vi "Test Configure device.vi"   [LabVIEW 2020]
uses:
  WS1051 1.1/WS1051 1.1.lvclass
  C:/Sandbox/RF Bench/Source Code/WiSpry Test Framework/Devices/Toggle 7/Toggle 7.1.lvclass
  WS1050 1.1/WS1050 1.1.lvclass
  Controls/Change setting mode enum.ctl
  Toggle 7.1.lvclass
  PIC-device/PIC-Device.lvclass
types:
  T1 = typedef "PIC-Device.lvclass/Change setting mode enum.ctl" = enum16{"Init", "Next", "Reset"}
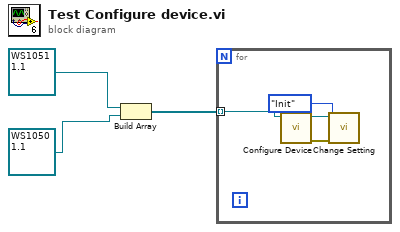
[diagram p0: block diagram]
diagram:
  n1 = Build Array(refnum<class "WS1051 1.1.lvclass"> refnum ("WS1051 1.1.lvclass"), refnum<class "WS1050 1.1.lvclass"> refnum ("WS1050 1.1.lvclass")) -> (w1:refnum<class "Toggle 7.1.lvclass">[])
  n2 = for {
    tunnel: w1 -> [w7] mode=indexing
    n3 = call-dynamic "Configure Device.vi"("Toggle 7 1.1 in"=w7) -> ("error out"=w5:errorcluster, "Toggle 7 1.1 out"=w6:refnum<class "Toggle 7.1.lvclass">)  [unwired: 9 in]
    n4 = call-dynamic "Change Setting.vi"("error in (no error)"=w5, "Change setting mode"=Change_setting_mode_enum."Init", "Toggle 6 in"=w6) -> ()  [unwired: 5 in, 4 out]
  }
